vi "Autonomous Play Execution concurrent.vi"(1 "Input Play":T2) -> (0 "Robot System Functions":T1)   [LabVIEW 2014]
uses:
  Autonomous Play Definition.ctl
  Autonomous Commands/Autonomous Command Names.ctl
  Subsystems VIs/Robot Commands.ctl
  Autonomous Play State.ctl
  Autonomous State global.vi
panel:
  # "Field Centric"
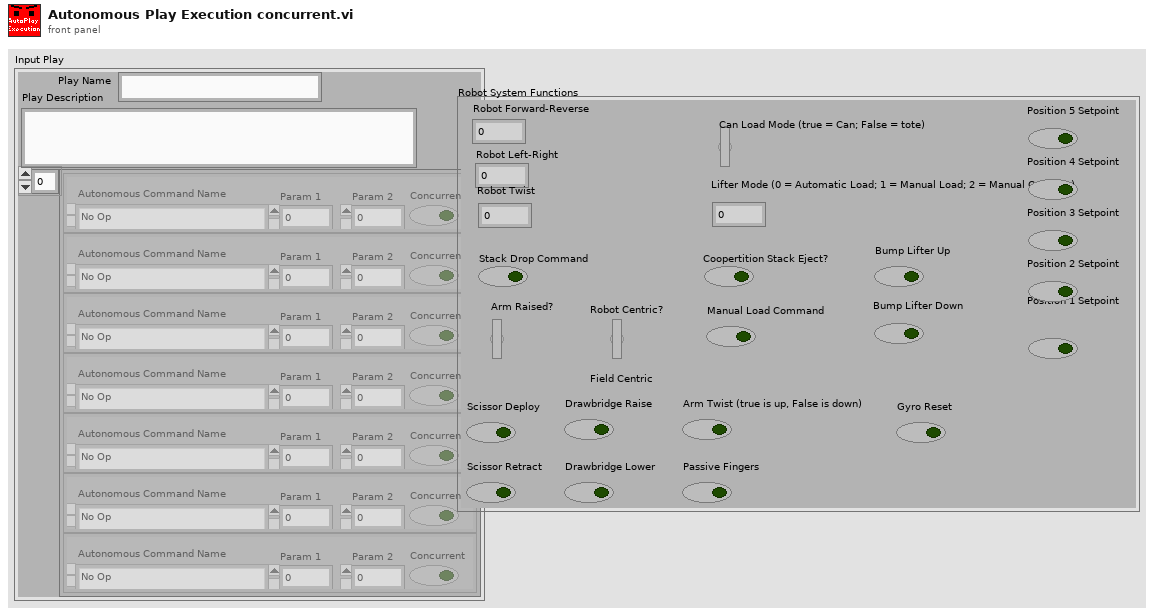
[diagram p1: front panel]
types:
  T1 = typedef "Robot Commands.ctl" = cluster{"Robot Forward-Reverse":dbl, "Robot Left-Right":dbl, "Robot Twist":dbl, "Can Load Mode (true = Can; False = tote)":bool, "Lifter Mode (0 = Automatic Load; 1 = Manual Load; 2 = Manual Override)":dbl, "Stack Drop Command":bool, "Arm Raised?":bool, "Coopertition Stack Eject?":bool, "Position 1 Setpoint":bool, "Position 2 Setpoint":bool, "Position 3 Setpoint":bool, "Position 4 Setpoint":bool, "Position 5 Setpoint":bool, "Bump Lifter Down":bool, "Bump Lifter Up":bool, "Manual Load Command":bool, "Robot Centric?":bool, "Scissor Deploy":bool, "Drawbridge Lower":bool, "Scissor Retract":bool, "Passive Fingers":bool, "Drawbridge Raise":bool, "Arm Twist (true is up, False is down)":bool, "Gyro Reset":bool}
  T2 = typedef "Autonomous Play Definition.ctl" = cluster{"Play Name":string, "Command List":cluster{"Param 1":dbl, "Param 2":dbl, "Autonomous Command Name":T3, "Concurrent":bool}[], "Play Description":string}
  T3 = typedef "Autonomous Command Names.ctl" = enum16{"No Op", "Move Forward-Backward", "Translate Left-Right"}
  T4 = typedef "Autonomous Play State.ctl" = cluster{"Play Name":string, "Autonomous Command Name":T3, "Param 1":dbl, "Param 2":dbl, "Cmd Counter":i32, "Completed":bool}
  T5 = cluster{"Param 1":dbl, "Param 2":dbl, "Autonomous Command Name":T3, "Concurrent":bool}[]
  T6 = cluster{"Param 1":dbl, "Param 2":dbl, "Autonomous Command Name":T3, "Concurrent":bool}
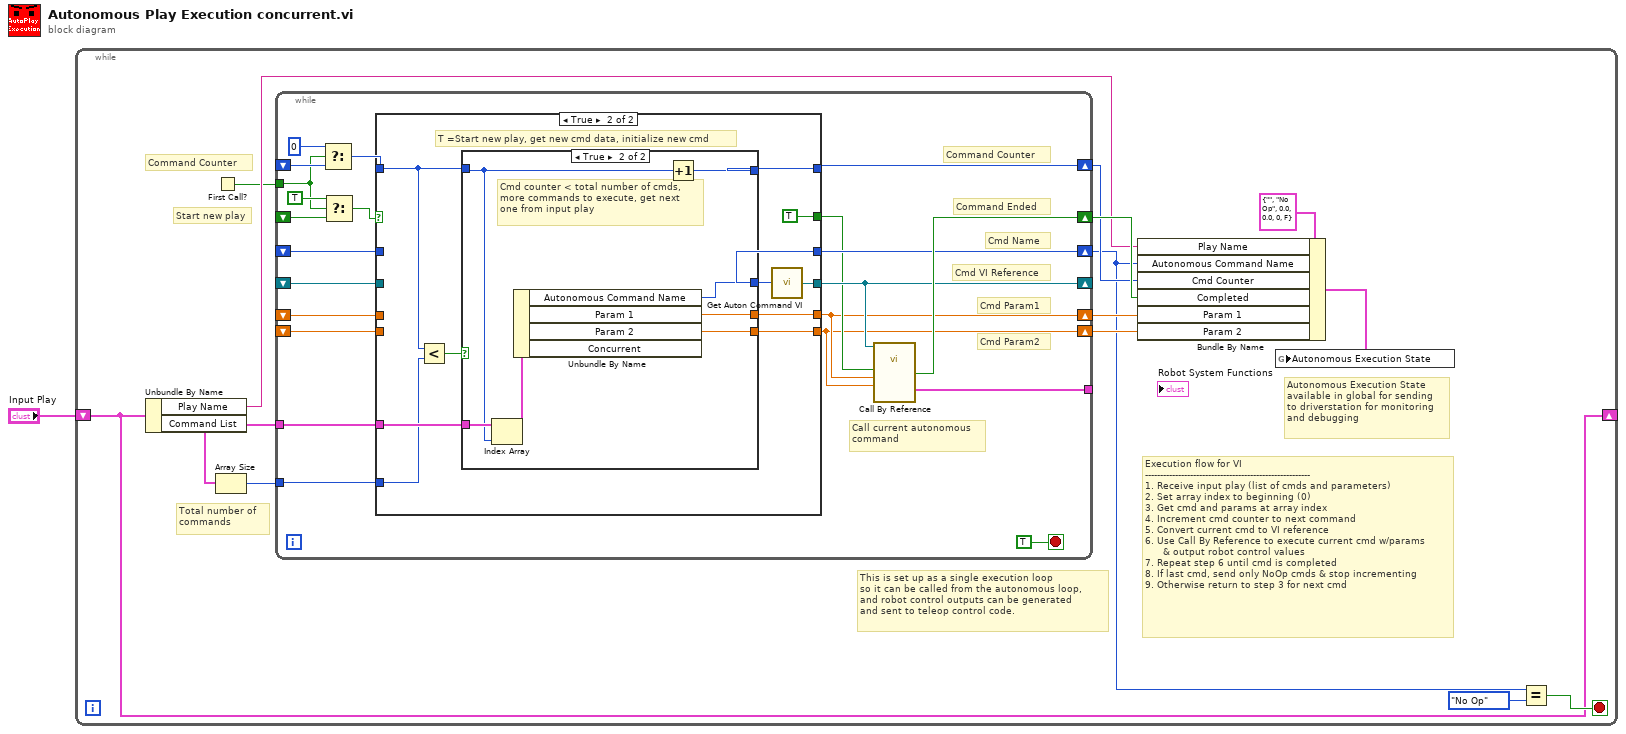
[diagram p0: block diagram]
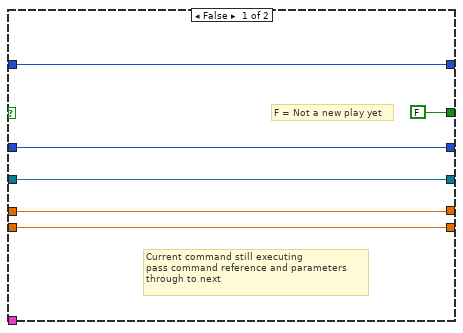
[diagram p2: hidden frame]
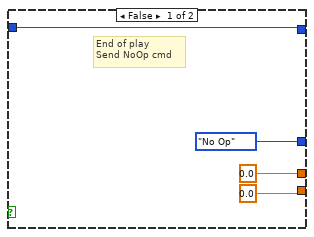
[diagram p3: hidden frame]
diagram:
  n1 = while {
    shift-right: [w2] -> _
    shift-left: "Input Play" -> [w2]
    stop <- w3 stop-if-true
    # "Autonomous Execution State\navailable in global for sending\nto driverstation for monitoring\nand debugging"
    # "This is set up as a single execution loop\nso it can be called from the autonomous loop, \nand robot control outputs can be generated \nand sent to teleop control code."
    # "Execution flow for VI\n-------------------------------------------------------\n1. Receive input play (list of cmds and parameters)\n2. Set array index to beginning (0)\n3. Get cmd and params at array index\n4. Increment cmd counter to next command\n5. Convert current cmd to VI reference\n6. Use Call By Reference to execute current cmd w/params\n      & output robot control values\n7. Repeat step 6 until cmd is completed\n8. If last cmd, send only NoOp cmds & stop incrementing \n9. Otherwise return to step 3 for next cmd"
    # "Start new play"
    # "Total number of \ncommands"
    # "Command Counter"
    n2 = Unbundle By Name(w2) -> ("Play Name"=w7:string, "Command List"=w8:T5)
    n3 = First Call?() -> (First Call?: T/F=w6:bool)
    n4 = Array Size(array=w8) -> (size(s)=w15:i32)
    n5 = while {
      tunnel: w8 -> [w37]
      tunnel: w15 -> [w29]
      shift-right: [w35] -> w9
      shift-left: _ -> [w24]
      shift-right: [w36] -> w10
      shift-left: _ -> [w22]
      shift-right: [w17] -> w12
      shift-left: _ -> [w33]
      shift-right: [w19] -> _
      shift-left: _ -> [w34]
      shift-right: [w16] -> w11
      shift-left: _ -> [w32]
      tunnel: [w31] -> _
      shift-right: [w28] -> w5
      shift-left: _ -> [w27]
      tunnel: w6 -> [w20]
      stop <- TRUE stop-if-true
      # "Cmd Name"
      # "Cmd Param2"
      # "Cmd Param1"
      # "Cmd VI Reference"
      # "Command Ended"
      # "Command Counter"
      # "Call current autonomous\ncommand"
      n6 = Select(t=0, s=w20, f=w24) -> (s? t:f=w25:i32)
      n7 = Select(t=TRUE, s=w20, f=w22) -> (s? t:f=w26:bool)
      n8 = case shown="True" w26 {
        tunnel: w37 -> [_ w53]
        tunnel: w25 -> [w43 w47]
        tunnel: [w40 w52] -> w16
        tunnel: [w41 w51] -> w17
        tunnel: [w38 w50] -> w19
        tunnel: [w43 w45] -> w35
        tunnel: [FALSE TRUE] -> w18
        tunnel: w34 -> [w38 _]
        tunnel: w33 -> [w41 _]
        tunnel: w32 -> [w40 _]
        tunnel: w29 -> [_ w46]
        tunnel: [w39 w44] -> w28
        tunnel: w27 -> [w39 _]
        frame False {
          # "F = Not a new play yet"
          # "Current command still executing\npass command reference and parameters \nthrough to next"
        }
        frame True {
          # "T =Start new play, get new cmd data, initialize new cmd"
          n9 = Less?(x=w47, y=w46) -> (x < y?=w48:bool)
          n10 = case shown="True" w48 {
            tunnel: w53 -> [_ w64]
            tunnel: [0.0 ("Param 2") w62] -> w52
            tunnel: [0.0 ("Param 1") w61] -> w51
            tunnel: w47 -> [w55 w60]
            tunnel: [w55 w59] -> w45
            tunnel: [Autonomous_Command_Names."No Op" ("Autonomous Command Name") w58] -> w44
            frame False {
              # "End of play\nSend NoOp cmd"
            }
            frame True {
              # "Cmd counter < total number of cmds,\nmore commands to execute, get next\none from input play"
              n11 = Index Array(array=w64, index=w60) -> (element=w63:T6)
              n12 = Unbundle By Name(w63) -> ("Autonomous Command Name"=w58:T3, "Param 1"=w61:dbl, "Param 2"=w62:dbl)  [unwired: 1 out]
              n13 = Increment(x=w60) -> (x+1=w59:i32)
            }
          }
          n14 = call "Get Auton Command VI.vi"("Autonomous Command Name"=w44) -> ("VI Refnum"=w50:refnum<vi>)
        }
      }
      n15 = call-by-ref "?"(reference=w19, "Cmd Parameter 1"=w16, "Cmd Parameter 2"=w17, "Startup"=w18) -> ("Robot System Functions"=w31:T1, "Completed"=w36:bool)  [unwired: 2 in, 2 out]
    }
    n16 = Bundle By Name(cluster=T4 {"Play Name"="", "Autonomous Command Name"=enum."No Op", "Param 1"=0.0, "Param 2"=0.0, "Cmd Counter"=0, "Completed"=FALSE} ("Autonomous Execution State"), "Play Name"=w7, "Autonomous Command Name"=w5, "Cmd Counter"=w9, "Completed"=w10, "Param 1"=w12, "Param 2"=w11) -> (w13:T4)
    n17 = global write "Autonomous State global.vi" "Autonomous Execution State"(w13) -> ()
    n18 = Equal?(x=w5, y=Autonomous_Command_Names."No Op") -> (x = y?=w3:bool)
  }
